vi "SUB_VI_scrittura_messaggio.vi"(8 "Errore in ingresso":errorcluster, 10 "Messaggio da inviare":string, 11 "TCP Network \nConnection in":refnum<k5>) -> (0 "Errore in uscita":errorcluster, 3 "TCP Network \nConnection out":refnum<k5>)   [LabVIEW 2023]
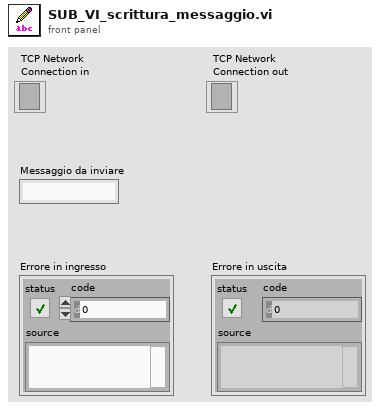
[diagram p1: front panel]
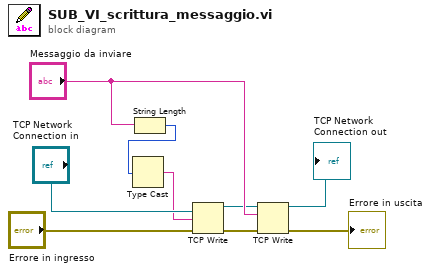
[diagram p0: block diagram]
diagram:
  n1 = String Length(string="Messaggio da inviare") -> (length=w1:i32)
  n2 = Type Cast(x=w1) -> (*(type *) &x=w2:string)  [unwired: 1 in]
  n3 = TCP Write(connection ID="TCP Network \nConnection in", data in=w2, error in (no error)="Errore in ingresso") -> (connection ID out=w3:refnum<k5>, error out=w4:errorcluster)  [unwired: 1 in, 1 out]
  n4 = TCP Write(connection ID=w3, data in="Messaggio da inviare", error in (no error)=w4) -> (connection ID out=→"TCP Network \nConnection out":refnum<k5>, error out=→"Errore in uscita":errorcluster)  [unwired: 1 in, 1 out]
